vi "Create ModSweep Evals.vi"(8 "error in (no error)":errorcluster, 11 "ModSweep in":refnum<class "ModSweep.lvclass">) -> (0 "error out":errorcluster, 2 "Array":T1[](array[typedef]) {"Low Limit" format="%#_13g"; "SI Scaling" items=["femto"=-15, "pico"=-12, "nano"=-9, "micro"=-6, "milli"=-3, "percent"=-2, ""=0, "kilo"=3, "mega"=6, "giga"=9, "tera"=12]}, 3 "ModSweep out":refnum<class "ModSweep.lvclass">)   [LabVIEW 2018, in "ModSweep.lvlib" / "ModSweep.lvclass"]
uses:
  ModSweep.lvclass
  Plugins/TestStand API Tools (TSAT).lvlibp/Evaluation Actions/Includes/Controls/TSAT Evaluation.ctl
  Plugins/TestStand API Tools (TSAT).lvlibp/Evaluation Actions/TSAT Evaluation Actions.lvlib
  Plugins/String Database.lvlibp/String Database.lvclass
  Plugins/Test Number and Bin Generator.lvlibp/Test Number and Bin Generator/Test Number and Bin Generator.lvclass
  Plugins/TestStand API Tools (TSAT).lvlibp/Evaluation Actions/Includes/Controls/TSAT Eval SI Unit Scaling.ctl
  Plugins/SeqAuto Evaluations.lvlibp/ModSweep/ModSweep Gain/ModSweep Gain.lvclass
  Plugins/TestStand API Tools (TSAT).lvlibp/Evaluation Actions/Includes/Controls/TSAT Evaluation Type.ctl
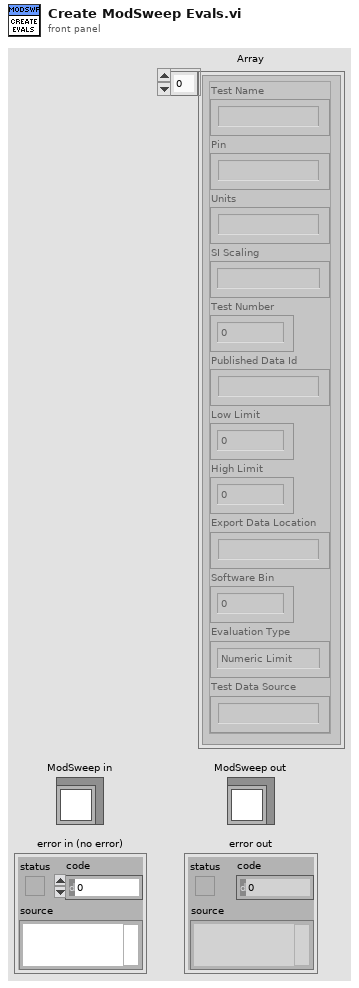
[diagram p1: front panel]
types:
  T1 = typedef "TestStand API Tools (TSAT).lvlibp/TSAT Evaluation Actions.lvlib/TSAT Evaluation.ctl" = cluster{"Test Name":string, "Pin":string, "Units":string, "SI Scaling":T2, "Test Number":i32, "Published Data Id":string, "Low Limit":dbl, "High Limit":dbl, "Export Data Location":string, "Software Bin":i64, "Evaluation Type":T3, "Test Data Source":string}
  T2 = typedef "TestStand API Tools (TSAT).lvlibp/TSAT Evaluation Actions.lvlib/TSAT Eval SI Unit Scaling.ctl" = i16
  T3 = typedef "TestStand API Tools (TSAT).lvlibp/TSAT Evaluation Actions.lvlib/TSAT Evaluation Type.ctl" = enum16{"Numeric Limit", "Pass/Fail", "None"}
  T4 = typedef "Test Number and Bin Generator.lvlibp/Test Number and Bin Generator.lvclass/Session Handle.ctl" = refnum<data-value>
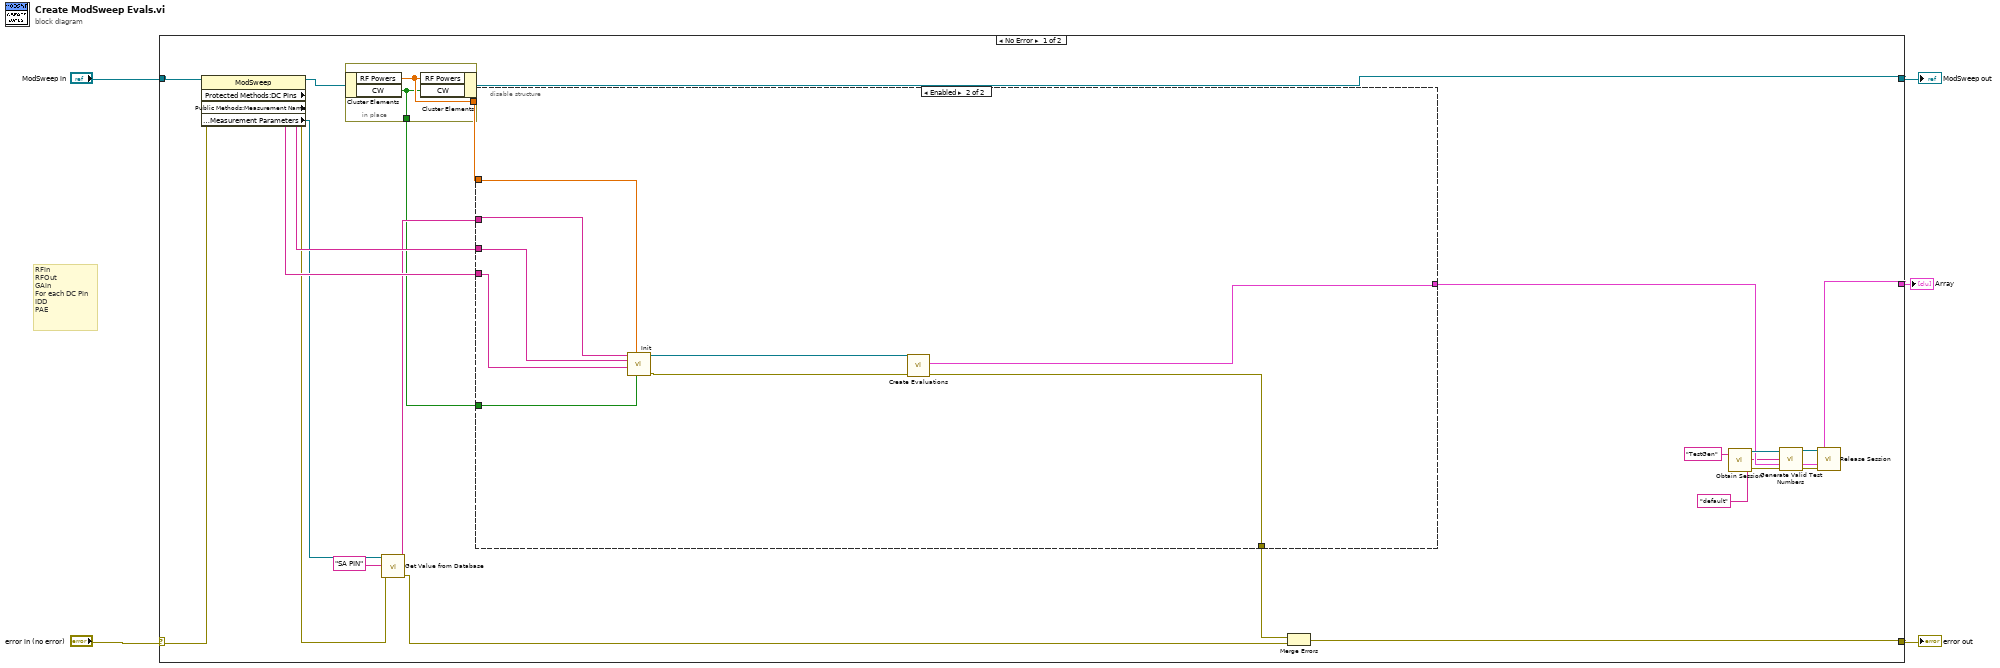
[diagram p0: block diagram]
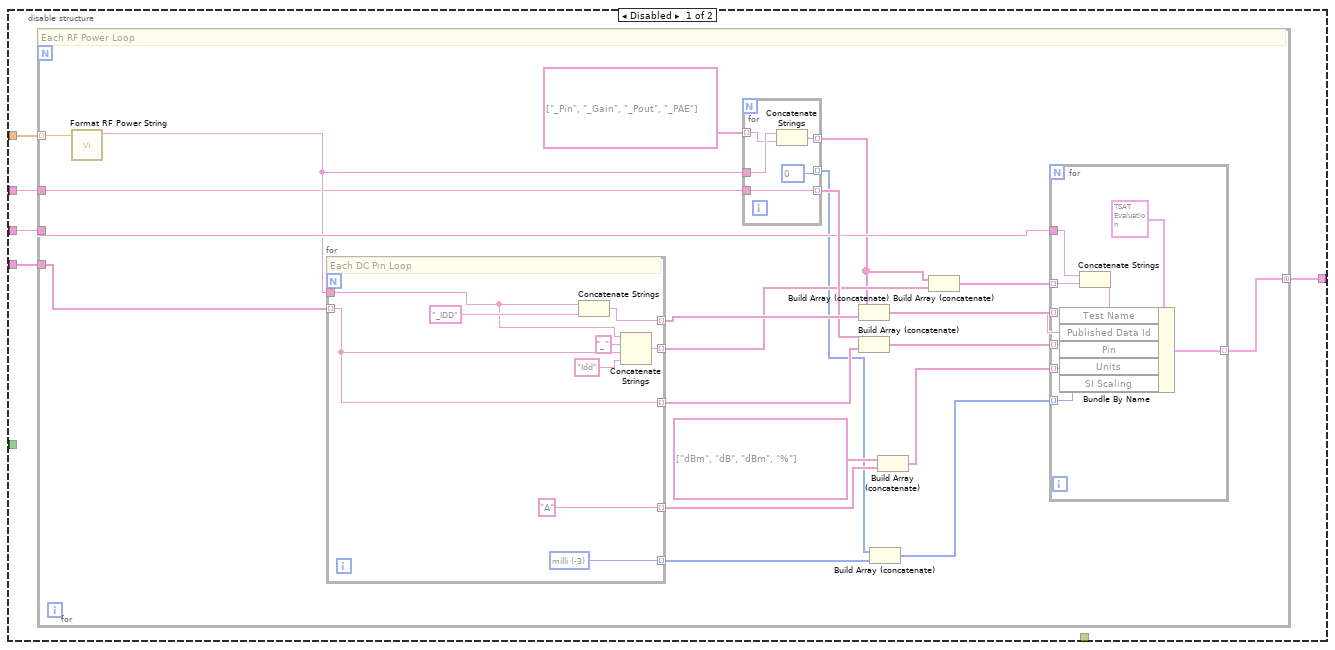
[diagram p2: hidden frame]
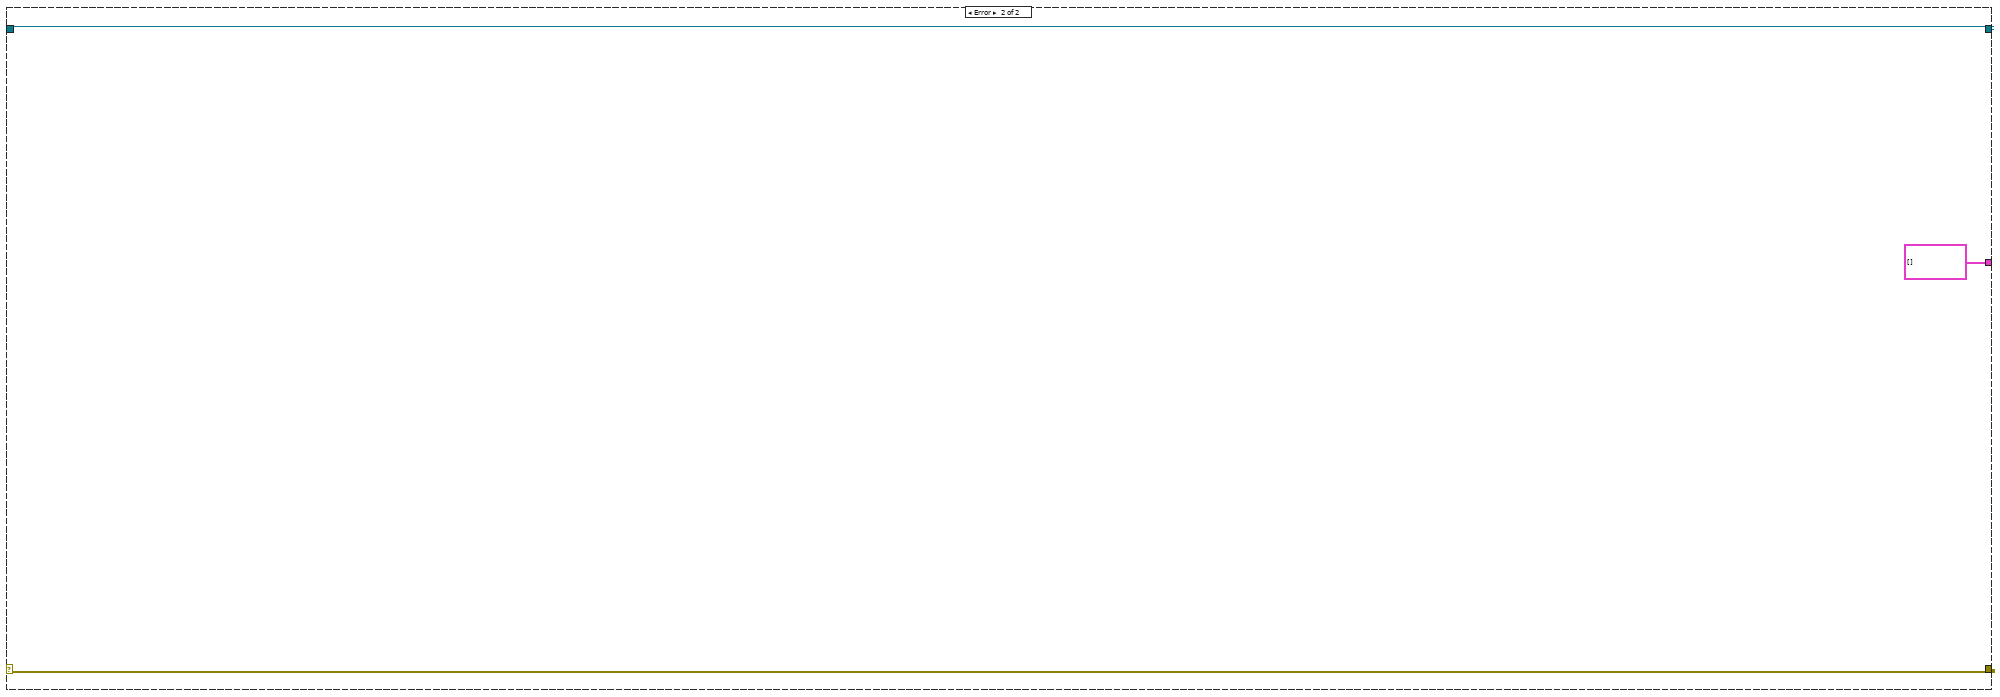
[diagram p3: hidden frame]
diagram:
  # "RFin\nRFOut\nGAin\nFor each DC Pin\nIDD\nPAE"
  n1 = case shown="No Error" "error in (no error)" {
    selector: "error in (no error)" -> [w28 w91]
    tunnel: [w9 w91] -> w4
    tunnel: [w25 w90] -> w2
    tunnel: "ModSweep in" -> [w27 w90]
    tunnel: [w11 T1[] []] -> w1
    frame No Error {
      n2 = property class="ModSweep"(reference=w27, error in=w28) -> (reference out=w26:refnum<class "ModSweep.lvclass">, error out=w20:errorcluster, "Protected Methods:DC Pins"=w23:string[], "Public Methods:Measurement Name"=w22:string, "Protected Methods:Measurement Parameters"=w21:refnum<class "String Database.lvclass">)
      n3 = in-place {
        in-place-border: [w88] -> w24
        in-place-border: [w87] -> w7
        n4 = in-place-cluster #1(w26) -> ("RF Powers"=w88:dbl[], "CW"=w87:bool)
        n5 = in-place-cluster #1("RF Powers"=w88, "CW"=w87) -> (w25:refnum<class "ModSweep.lvclass">)
      }
      n6 = call "Get Value from Database.vi"("error in (no error)"=w20, "Entry Name"="SA PIN", "Message in"=w21) -> ("error out"=w18:errorcluster, "Entry Value"=w17:string)  [unwired: 5 in, 2 out]
      n7 = disable-structure shown="Enabled" {
        disable-tunnel: w24 -> [w33 w84]
        disable-tunnel: w23 -> [w32 w81]
        disable-tunnel: w17 -> [w31 w82]
        disable-tunnel: w22 -> [w30 w83]
        disable-tunnel: [w29 w80] -> w10
        disable-tunnel: [_ w79] -> w8
        disable-tunnel: w7 -> [_ w78]
        frame Disabled {
          n8 = for {
            tunnel: w33 -> [w36] mode=indexing
            tunnel: w32 -> [w46]
            tunnel: w30 -> [w48]
            tunnel: w31 -> [w34]
            tunnel: [w47] -> w29 mode=concatenating
            # "Each RF Power Loop"
            n9 = call "Format RF Power String.vi"("x"=w36) -> ("result string"=w35:string)  [unwired: 10 in]
            n10 = for {
              tunnel: w35 -> [w69]
              tunnel: [w76] -> w53 mode=indexing
              tunnel: [w72] -> w50 mode=indexing
              tunnel: w46 -> [w72] mode=indexing
              tunnel: ["A"] -> w44 mode=indexing
              tunnel: [w75] -> w42 mode=indexing
              tunnel: [w74] -> w38 mode=indexing
              w74 = T2 -3 items=["femto"=-15, "pico"=-12, "nano"=-9, "micro"=-6, "milli"=-3, "percent"=-2, ""=0, "kilo"=3, "mega"=6, "giga"=9, "tera"=12] ("SI Scaling")
              # "Each DC Pin Loop"
              n11 = Concatenate Strings(w69, "_IDD" ("string")) -> (w76:string)
              n12 = Concatenate Strings(w69, "_" ("string"), w72, "Idd" ("string")) -> (w75:string)
            }
            n13 = for {
              tunnel: string[] ["_Pin", "_Gain", "_Pout", "_PAE"] -> [w65] mode=indexing
              tunnel: w35 -> [w66]
              tunnel: [w68] -> w41 mode=indexing
              tunnel: [w67] -> w51 mode=indexing
              tunnel: w34 -> [w67]
              tunnel: [w64] -> w39 mode=indexing
              w64 = T2 0 items=["femto"=-15, "pico"=-12, "nano"=-9, "micro"=-6, "milli"=-3, "percent"=-2, ""=0, "kilo"=3, "mega"=6, "giga"=9, "tera"=12] ("SI Scaling")
              n14 = Concatenate Strings(w66, w65) -> (w68:string)
            }
            n15 = Build Array (concatenate)(w41, w53) -> (w52:string[])
            n16 = Build Array (concatenate)(w51, w50) -> (w49:string[])
            n17 = Build Array (concatenate)(w39, w38) -> (w37:T2[])
            n18 = Build Array (concatenate)(string[] ["dBm", "dB", "dBm", "%"], w44) -> (w43:string[])
            n19 = Build Array (concatenate)(w41, w42) -> (w40:string[])
            n20 = for {
              tunnel: w52 -> [w61] mode=indexing
              tunnel: w49 -> [w63] mode=indexing
              tunnel: w43 -> [w62] mode=indexing
              tunnel: w48 -> [w57]
              tunnel: [w59] -> w47 mode=indexing
              tunnel: w40 -> [w58] mode=indexing
              tunnel: w37 -> [w55] mode=indexing
              n21 = Concatenate Strings(w57, w58) -> (w56:string)
              n22 = Bundle By Name(cluster=T1 {"Test Name"="", "Pin"="", "Units"="", "SI Scaling"=0, "Test Number"=0, "Published Data Id"="", "Low Limit"=-999999.0, "High Limit"=999999.0, "Export Data Location"="", "Software Bin"=-1, "Evaluation Type"=enum."Numeric Limit", "Test Data Source"=""} ("Evaluation"), "Test Name"=w56, "Published Data Id"=w61, "Pin"=w63, "Units"=w62, "SI Scaling"=w55) -> (w59:T1)
            }
          }
        }
        frame Enabled {
          n23 = call "Init.vi"("CW?"=w78, "RF Powers"=w84, "DC Pins"=w81, "Measurement Name"=w83, "SA Pin"=w82) -> ("error out"=w85:errorcluster, "ModSweep Gain out"=w86:refnum<class "ModSweep Gain.lvclass">)  [unwired: 5 in]
          n24 = call-dynamic "Create Evaluations.vi"("error in (no error)"=w85, "IEvaluation in"=w86) -> ("error out"=w79:errorcluster, "Evaluations Out"=w80:T1[])  [unwired: 7 in, 1 out]
        }
      }
      n25 = Merge Errors(w8, w18) -> (w9:errorcluster)
      n26 = call "Obtain Session.vi"("Session  Name ()"="TestGen") -> ("Session Handle"=w13:T4, "error out"=w14:errorcluster)  [unwired: 13 in]
      n27 = call "Generate Valid Test Numbers.vi"("Session Handle in"=w13, "Test Group"="default", "Evaluations In"=w10, "error in (no error)"=w14) -> ("Session Handle out"=w15:T4, "Evaluations Out"=w11:T1[], "error out"=w16:errorcluster)  [unwired: 9 in]
      n28 = call "Release Session.vi"("Session Handle"=w15, "error in (no error)"=w16) -> ()  [unwired: 13 in, 1 out]
    }
    frame Error {
    }
  }
  "error out" <- w4
  "ModSweep out" <- w2
  "Array" <- w1
